vi "CallBack Change Data Type.vi"(6 "Variant":variant, 8 "error in (no error)":errorcluster, 9 "old values":string[][](array[string]), 10 "object ref in":T2, 11 "Cluster":T3) -> (0 "error out":errorcluster)   [LabVIEW 2013, in "Modbus Module editor node.lvclass"]
uses:
  Modbus Module editor node.lvclass
  <vilib>/NI/DCAF Table API/Table Manager/Cell Change.ctl
  <vilib>/NI/DCAF Table API/Table Manager/object ref.ctl
  <vilib>/NI/DCAF/Tag Editor Core/Configuration Editor/Classes/Engine Parent/Engine Parent Editor Node.lvclass
  <vilib>/NI/DCAF/Tag Editor Core/Configuration Editor/Classes/Module editor node/module editor node.lvclass
  <vilib>/NI/Tag Bus/tag/Data Type.ctl
  module/configuration/Modbus Module configuration.lvclass
  <vilib>/NI/Configuration Framework/serializable configuration/NISE_CEF_serializable configuration.lvclass/NISE_CEF_serializable configuration.ctl
  <vilib>/NI/Tag Bus/tag/tag descriptor.lvclass/tag descriptor.ctl
  <vilib>/Utility/LVClass/Get LV Class Name.vi
  <vilib>/NI/Configuration Framework/error generator/NISE_error generator.vi
  <vilib>/NI/Tag Bus/tag/tag descriptor.lvclass
  <vilib>/NI/Configuration Framework/serializable configuration/NISE_CEF_serializable configuration.lvclass
  <vilib>/NI/DCAF Table API/Table Manager.lvlib
  <vilib>/NI/Module Execution Interface/Engine Configuration/engine configuration.lvclass
  <vilib>/NI/DCAF Table API/Table Manager/Table Manager.lvclass
panel:
  in  "data type":T1
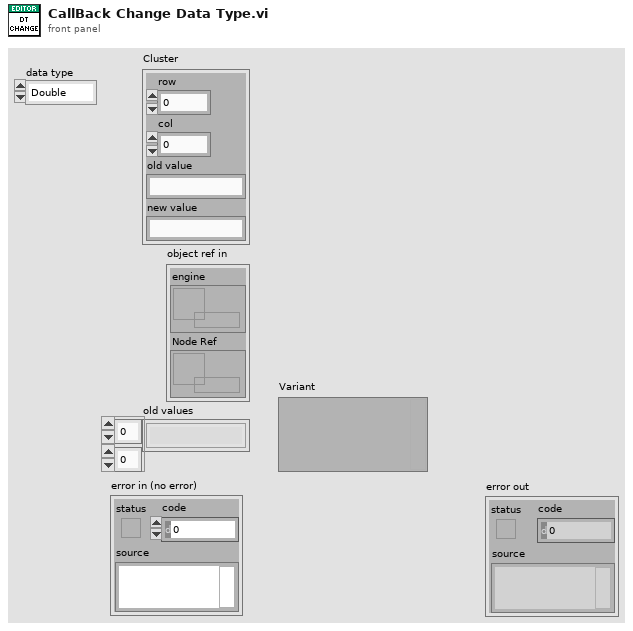
[diagram p1: front panel]
types:
  T1 = typedef "tag bus.lvlib/tag descriptor.lvclass/Data Type.ctl" = enum16{"Double", "Single", "I64", "I32", "I16", "I8", "U64", "U32", "U16", "U8", "Boolean", "String", "Array of Double", "Array of Single", "Array of I64", "Array of I32", "Array of I16", "Array of I8", "Array of U64", "Array of U32", "Array of U16", "Array of U8", "Array of Boolean", "Array of String"}
  T2 = typedef "Table Manager.lvlib/Table Manager.lvclass/object ref.ctl" = cluster{"engine":refnum<data-value>, "Node Ref":refnum<data-value>}
  T3 = typedef "Table Manager.lvlib/Cell Change.ctl" = cluster{"row":i32, "col":i32, "old value":string, "new value":string}
  T4 = typedef "Modbus Module configuration.lvclass/Line.ctl" = cluster{"MB Channel":refnum<class "Modbus Module Channel.lvclass">}
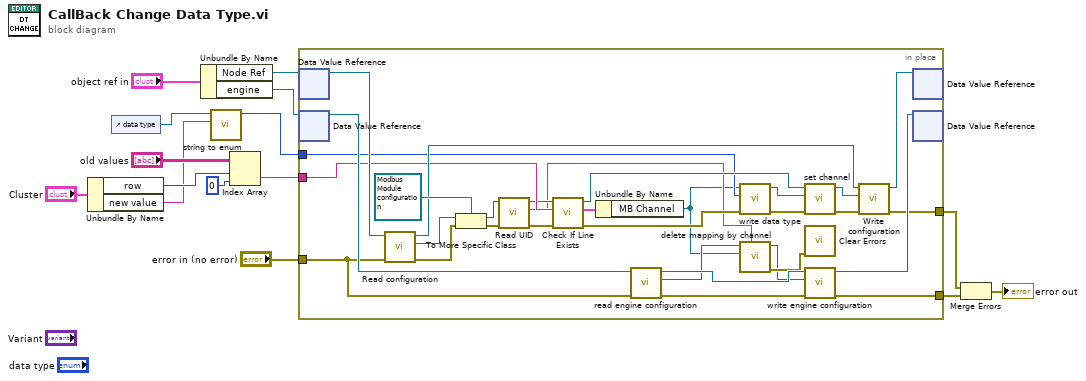
[diagram p0: block diagram]
diagram:
  n1 = Unbundle By Name("Cluster") -> ("row"=w11:i32, "new value"=w2:string)
  n2 = control-ref of="data type"() -> (w3:refnum<vi>)
  n3 = Unbundle By Name("object ref in") -> ("Node Ref"=w13:refnum<data-value>, "engine"=w12:refnum<data-value>)
  n4 = call <vilib>:"string to enum.vi"("String"=w2, "Enum"=w3) -> ("Value"=w1:i32)  [unwired: 8 in, 1 out]
  n5 = Index Array(array="old values", index (row)=w11, index (col)=0 ("disabled index (col)")) -> (element=w9:string)
  n6 = in-place {
    in-place-border: w9 -> [w38]
    in-place-border: "error in (no error)" -> [w20]
    in-place-border: [w22] -> w5
    in-place-border: [w21] -> w4
    in-place-border: w1 -> [w18]
    n7 = in-place-dvr #1(w13) -> (w43:refnum<class "module editor node.lvclass">)  [unwired: 1 out]
    n8 = in-place-dvr #2(w12) -> (w39:refnum<class "Engine Parent Editor Node.lvclass">)  [unwired: 1 out]
    n9 = call-dynamic "Read configuration.vi"("error in"=w20, "NISE_CEF_serializable node in"=w43) -> ("error out"=w23:errorcluster, "configuration"=w45:refnum<class "NISE_CEF_serializable configuration.lvclass">, "NISE_CEF_serializable node out"=w42:refnum<class "module editor node.lvclass">)  [unwired: 7 in]
    n10 = To More Specific Class(target class=refnum<class "Modbus Module configuration.lvclass"> refnum ("Modbus Slave configuration in"), reference=w45, error in=w23) -> (specific class reference=w33:refnum<class "Modbus Module configuration.lvclass">, error out=w27:errorcluster)
    n11 = call <vilib>:"Read UID.vi"("error in"=w27, "configuration in"=w33) -> ("error out"=w26:errorcluster, "instance id"=w31:string, "configuration out"=w32:refnum<class "Modbus Module configuration.lvclass">)  [unwired: 7 in]
    n12 = call "Check If Line Exists.vi"("error in (no error)"=w26, "Name to locate"=w38, "Modbus Slave configuration in"=w32) -> ("error out"=w37:errorcluster, "Line out"=w17:T4, "Modbus Slave configuration out"=w36:refnum<class "Modbus Module configuration.lvclass">)  [unwired: 4 in, 2 out]
    n13 = Unbundle By Name(w17) -> ("MB Channel"=w16:refnum<class "Modbus Module Channel.lvclass">)
    n14 = call <vilib>:"read engine configuration.vi"("error in"=w20, "Engine Parent Editor Node in"=w39) -> ("error out"=w19:errorcluster, "engine configuration"=w28:refnum<class "engine configuration.lvclass">, "Engine Parent Editor Node out"=w40:refnum<class "Engine Parent Editor Node.lvclass">)  [unwired: 7 in]
    n15 = call <vilib>:"write data type.vi"("error in"=w37, "data type"=w18, "system tag in"=w16) -> ("error out"=w25:errorcluster, "system tag out"=w35:refnum<class "Modbus Module Channel.lvclass">)  [unwired: 7 in]
    n16 = call <vilib>:"delete mapping by channel.vi"("owner ID"=w31, "channel"=w16, "engine configuration in"=w28) -> ("error out"=w30:errorcluster, "engine configuration out"=w29:refnum<class "engine configuration.lvclass">)  [unwired: 7 in]
    n17 = call "set channel.vi"("error in"=w25, "Modbus Module Channel.lvclass"=w35, "Modbus Slave configuration in"=w36) -> ("error out"=w24:errorcluster, "Modbus Slave configuration out"=w34:refnum<class "Modbus Module configuration.lvclass">)  [unwired: 7 in]
    n18 = call <vilib>:"Clear Errors.vi"("error in (no error)"=w30) -> ()  [unwired: 6 in, 1 out]
    n19 = call <vilib>:"write engine configuration.vi"("error in"=w19, "engine configuration"=w29, "Engine Parent Editor Node in"=w40) -> ("error out"=w22:errorcluster, "Engine Parent Editor Node out"=w41:refnum<class "Engine Parent Editor Node.lvclass">)  [unwired: 7 in]
    n20 = call-dynamic "Write configuration.vi"("error in"=w24, "configuration"=w34, "NISE_CEF_serializable node in"=w42) -> ("error out"=w21:errorcluster, "NISE_CEF_serializable node out"=w44:refnum<class "module editor node.lvclass">)  [unwired: 7 in]
    n21 = in-place-dvr #1(w44) -> ()  [unwired: 2 out]
    n22 = in-place-dvr #2(w41) -> ()  [unwired: 2 out]
  }
  n23 = Merge Errors(w4, w5) -> (→"error out":errorcluster)
